vi "ZMC Find Next3File.vi"(8 "error in (no error)":errorcluster caption="错误输入（无错误）", 9 "pFileSize":u32, 10 "pfilenameinControl":string, 11 "handle":u32) -> (0 "error out":errorcluster caption="错误输出", 1 "pFileSize out":u32, 2 "pfilenameinControl out":string, 3 "handle out":u32, 5 "function return":i32)   [LabVIEW 2015, in "zauxdll.lvlib"]
doc: "int32 __stdcall ZMC_FindNext3File(ZMC_HANDLE handle, char* pfilenameinControl, uint32 *pFileSize);"
uses:
  zauxdll.lvlib
  zmotion.dll
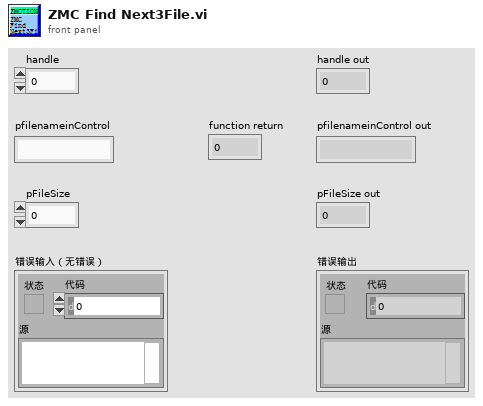
[diagram p1: front panel]
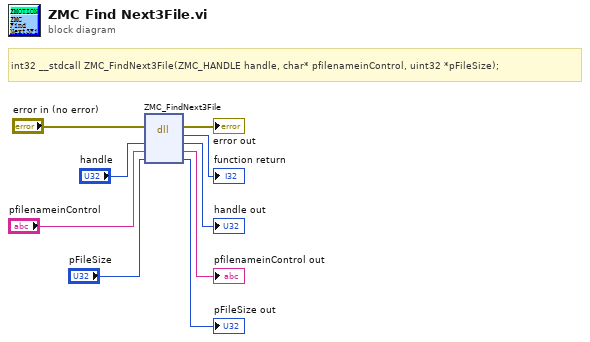
[diagram p0: block diagram]
diagram:
  # "int32 __stdcall ZMC_FindNext3File(ZMC_HANDLE handle, char* pfilenameinControl, uint32 *pFileSize);"
  n1 = dll-call lib="C:/Users/VIC/Desktop/GOGORO_SA/system/LLB/zmotion/zaux/zmotion.*" fn="ZMC_FindNext3File"(error in="error in (no error)", "handle"="handle", "pfilenameinControl"="pfilenameinControl", "pFileSize"="pFileSize") -> (error out=→"error out":errorcluster, →"function return":i32, "handle"=→"handle out":u32, "pfilenameinControl"=→"pfilenameinControl out":string, "pFileSize"=→"pFileSize out":u32)  [unwired: 2 in, 1 out]
